vi "Default design values.vi"() -> (1 "label array":string[](array[string]), 2 "Array to save":cluster{"Label.Text":string, "Value":variant}[](array[cluster]), 3 "Input Cluster":T1={"Project Info"={"Project Name"="New Project", "City"="", "State"="", "Notes"=""}, "Basic Inputs"={"Q.Plant"=0.018000000000000002, "C.CoagDoseMax"=0.08, "C.CoagStock"=120.0, "Ti.CoagStock"=108000.0, "EN.DrillSeries"=enum."English", "EN.TubeSeries"=enum."English", "N.SedTanks"=3.0, "N.SedBaysEst"=2.0, "W.SedPlate"=1.0, "L.SedPlateSheet"=3.0, "T.SedPlate"=0.002, "T.PlantWall"=0.15, "H.FlocOption"=0.0, "T.FlocBaffleRigidH"=0.15, "T.ConcreteMin"=0.05, "T.SedWeir"=0.04, "T.FlocBaffleRigidV"=0.05}} {"Basic Inputs"."T.FlocBaffleRigidV" min=0.0 max=0.2 step=0.001 format="%#.1f"; "Basic Inputs"."T.SedWeir" min=0.001 max=0.2 step=0.001 format="%#.1f"; "Basic Inputs"."T.SedPlate" min=0.001 max=0.05 step=0.001 format="%#.1f"; "Basic Inputs"."T.FlocBaffleRigidH" min=0.0 max=0.2 step=0.001 format="%#.1f"; "Basic Inputs"."T.ConcreteMin" min=0.005 max=0.2 step=0.001 format="%#.1f"; "Basic Inputs"."L.SedPlateSheet" min=0.3 max=8.0 step=0.01 format="%#.1f"; "Basic Inputs"."N.SedBaysEst" min=1.0 max=20.0 step=1.0 format="%#.0f"; "Basic Inputs"."N.SedTanks" min=1.0 max=20.0 step=1.0 format="%#.0f"; "Basic Inputs"."Ti.CoagStock" min=43200.0 max=360000.0 step=3600.0 format="%#.1f"; "Basic Inputs"."H.FlocOption" min=0.5 max=4.0 step=0.01 format="%#.2f"; "Basic Inputs"."C.CoagStock" min=50.0 max=500.0 step=1.0 format="%#.0f"; "Basic Inputs"."C.CoagDoseMax" min=0.03 max=0.2 step=0.005 format="%#.0f"; "Basic Inputs"."Q.Plant" min=0.001 max=0.2 step=0.0001 format="%#.1f"; "Basic Inputs"."T.PlantWall" min=0.05 max=0.5 step=0.001 format="%#.1f"; "Basic Inputs"."W.SedPlate" min=0.5 max=3.0 step=0.001 format="%#.1f"})   [LabVIEW 2015, in "AguaClara Library.lvlib"]
uses:
  AguaClara Library.lvlib
  Input Cluster.ctl
  Project inputs.ctl
  Basic Inputs.ctl
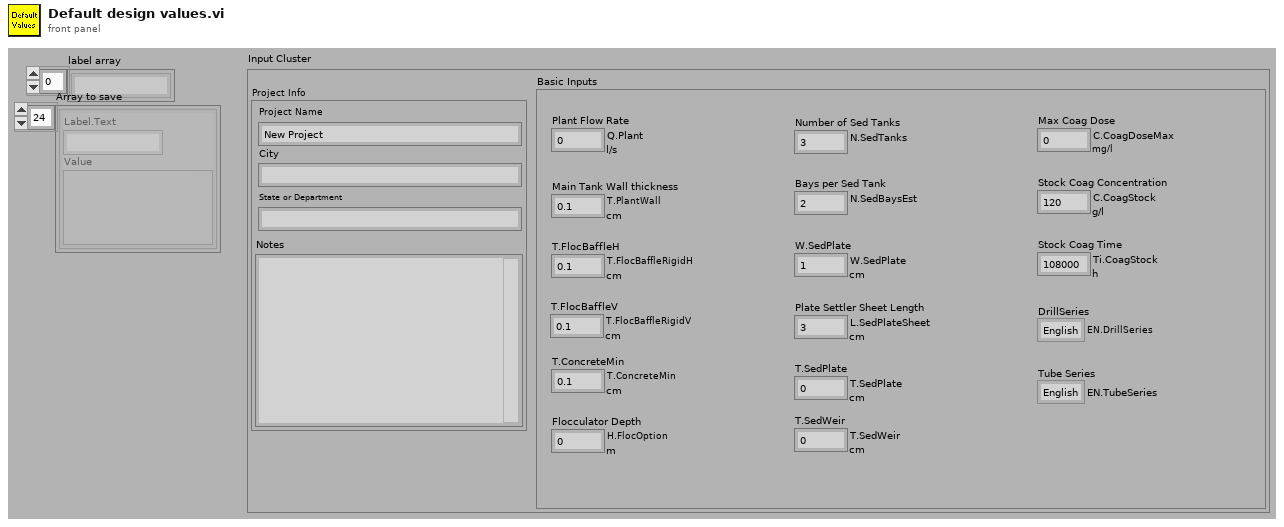
[diagram p1: front panel]
types:
  T1 = typedef "Input Cluster.ctl" = cluster{"Project Info":T2, "Basic Inputs":T3}
  T2 = typedef "AguaClara Library.lvlib/Project inputs.ctl" = cluster{"Project Name":string, "City":string, "State":string, "Notes":string}
  T3 = typedef "AguaClara Library.lvlib/Basic Inputs.ctl" = cluster{"Q.Plant":dbl[unit], "C.CoagDoseMax":dbl[unit], "C.CoagStock":dbl[unit], "Ti.CoagStock":dbl[unit], "EN.DrillSeries":enum16{"English", "Metric"}, "EN.TubeSeries":enum16{"English", "Metric"}, "N.SedTanks":dbl, "N.SedBaysEst":dbl, "W.SedPlate":dbl[unit], "L.SedPlateSheet":dbl[unit], "T.SedPlate":dbl[unit], "T.PlantWall":dbl[unit], "H.FlocOption":dbl[unit], "T.FlocBaffleRigidH":dbl[unit], "T.ConcreteMin":dbl[unit], "T.SedWeir":dbl[unit], "T.FlocBaffleRigidV":dbl[unit]}
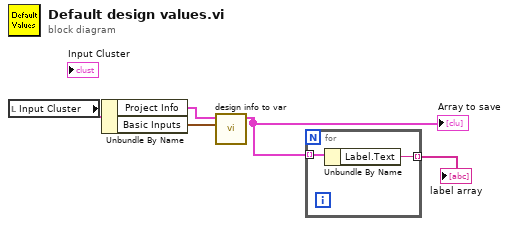
[diagram p0: block diagram]
diagram:
  n1 = local read "Input Cluster"() -> (w5:T1)
  n2 = Unbundle By Name(w5) -> ("Project Info"=w4:T2, "Basic Inputs"=w3:T3)
  n3 = call "design info to var.vi"("Design Inputs"=w3, "Project Info"=w4) -> ("Array to save"=w2:cluster{"Label.Text":string, "Value":variant}[])  [unwired: 9 in]
  "Array to save" <- w2
  n4 = for {
    tunnel: w2 -> [w7] mode=indexing
    tunnel: [w6] -> w1 mode=indexing
    n5 = Unbundle By Name(w7) -> ("Label.Text"=w6:string)
  }
  "label array" <- w1
